vi "Msg To Queue Actor.vi"(9 "Priority?":bool, 10 "Msg":refnum<class "Msg.lvclass">, 11 "jettl Event Actor in":refnum<class "jettl Event Actor.lvclass">) -> (0 "error out":errorcluster)   [LabVIEW 2021, in "jettl.lvlib" / "jettl Event Actor.lvlib" / "jettl Event Actor.lvclass"]
uses:
  jettl Event Actor.lvclass
  Actor/Msg/Msg.lvclass
  jettl Event Actor.lvclass/jettl Event Actor.ctl
  jettl.lvlib
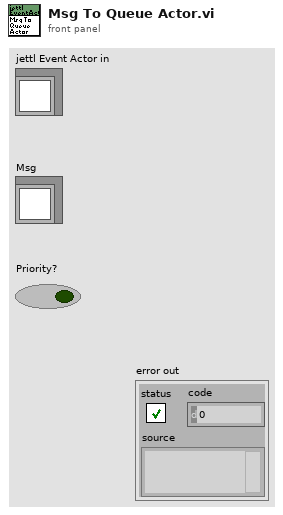
[diagram p1: front panel]
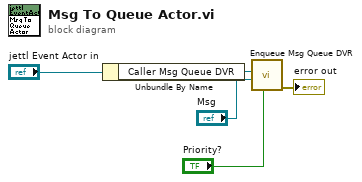
[diagram p0: block diagram]
diagram:
  n1 = Unbundle By Name("jettl Event Actor in") -> ("Caller Msg Queue DVR"=w4:refnum<data-value>)
  n2 = call "Enqueue Msg Queue DVR.vi"("Priority?"="Priority?", "Msg"="Msg", "Msg Queue DVR"=w4) -> ("error out"=→"error out":errorcluster)  [unwired: 8 in]
